vi "DI IRQ BuildMenu.vi"(0 "XRef":T15, 1 "MenuRef":T14, 2 "Point":T13, 3 "Menu Type":T12, 4 "State In":T2) -> (14 "Fatal Error Out":T1)   [LabVIEW 2021, in "myRIO Register DI IRQ.xnode"]
uses:
  <vilib>/myRIO/Instrument Drivers/IRQ/IO IRQ/vis/myRIO Register DI IRQ.xnode
  <vilib>/XNodeSupport/XNodeXNodeRef.ctl
  <vilib>/XNodeSupport/XNodeMenuRef.ctl
  <vilib>/XNodeSupport/XNodePoint.ctl
  <vilib>/XNodeSupport/XNodeInt.ctl
  <vilib>/XNodeSupport/XNodeMenuType.ctl
  <vilib>/myRIO/Instrument Drivers/IRQ/IO IRQ/vis/DI IRQ State.ctl
  <vilib>/myRIO/Common/Instrument Driver Framework/Utilities/typedefs/myRIOXPeripheral.ctl
  <vilib>/XNodeSupport/XNodeTerm4Array.ctl
  <vilib>/XNodeSupport/XNodeTerm4.ctl
  <vilib>/XNodeSupport/XNodeString.ctl
  <vilib>/XNodeSupport/XNodeVariant.ctl
  <vilib>/XNodeSupport/XNodeRect32.ctl
  <vilib>/XNodeSupport/XNodeBool.ctl
  <vilib>/XNodeSupport/XNodeTermDirection.ctl
  <vilib>/XNodeSupport/XNodeErrorCluster.ctl
  <vilib>/XNodeSupport/NI_XNodeSupport.lvlib
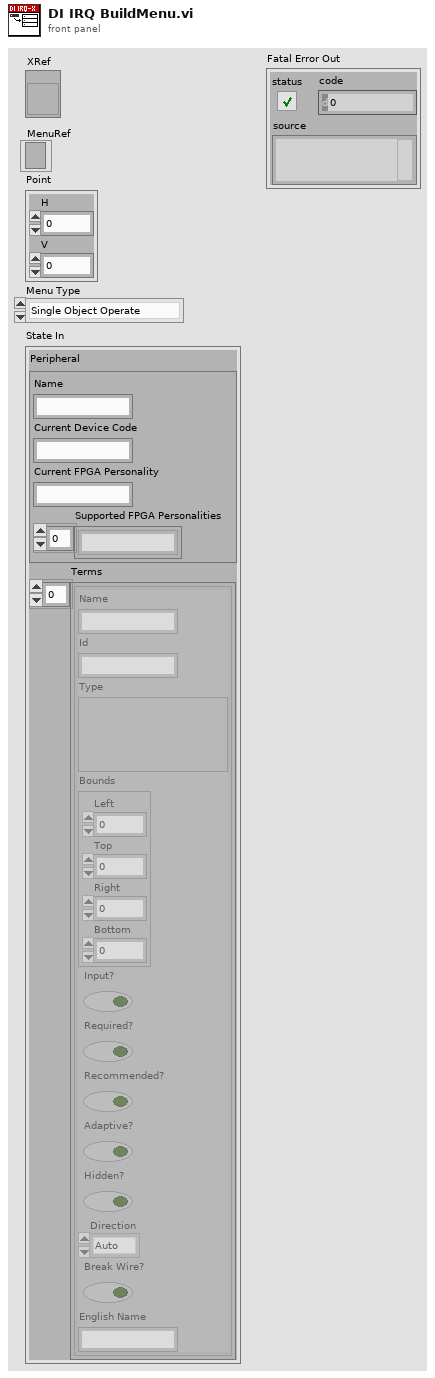
[diagram p1: front panel]
types:
  T1 = typedef "NI_XNodeSupport.lvlib/XNodeErrorCluster.ctl" = errorcluster
  T2 = typedef "myRIO Register DI IRQ.xnode/DI IRQ State.ctl" = cluster{"Peripheral":T3, "Terms":T4}
  T3 = typedef "myRIOXPeripheral.ctl" = cluster{"Name":string, "Current Device Code":string, "Current FPGA Personality":string, "Supported FPGA Personalities":string[]}
  T4 = typedef "NI_XNodeSupport.lvlib/XNodeTerm4Array.ctl" = T5[]
  T5 = typedef "NI_XNodeSupport.lvlib/XNodeTerm4.ctl" = cluster{"Name":T6, "Id":T6, "Type":T7, "Bounds":T8, "Input?":T10, "Required?":T10, "Recommended?":T10, "Adaptive?":T10, "Hidden?":T10, "Direction":T11, "Break Wire?":T10, "English Name":T6}
  T6 = typedef "NI_XNodeSupport.lvlib/XNodeString.ctl" = string
  T7 = typedef "NI_XNodeSupport.lvlib/XNodeVariant.ctl" = variant
  T8 = typedef "NI_XNodeSupport.lvlib/XNodeRect32.ctl" = cluster{"Left":T9, "Top":T9, "Right":T9, "Bottom":T9}
  T9 = typedef "NI_XNodeSupport.lvlib/XNodeInt.ctl" = i32
  T10 = typedef "NI_XNodeSupport.lvlib/XNodeBool.ctl" = bool
  T11 = typedef "NI_XNodeSupport.lvlib/XNodeTermDirection.ctl" = enum32{"Auto", "Up", "Down", "Left", "Right", "Center"}
  T12 = typedef "NI_XNodeSupport.lvlib/XNodeMenuType.ctl" = enum32{"Single Object Operate", "Single Object Popup", "Multi Object Popup Master", "Multi Object Popup Other"}
  T13 = typedef "NI_XNodeSupport.lvlib/XNodePoint.ctl" = cluster{"H":T9, "V":T9}
  T14 = typedef "NI_XNodeSupport.lvlib/XNodeMenuRef.ctl" = refnum<k9>
  T15 = typedef "NI_XNodeSupport.lvlib/XNodeXNodeRef.ctl" = refnum<vi>
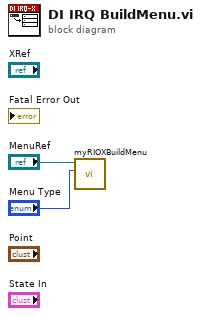
[diagram p0: block diagram]
diagram:
  n1 = call <vilib>:"myRIOXBuildMenu.vi"("Menu Type"="Menu Type", "Menu Reference"="MenuRef") -> ()  [unwired: 9 in, 1 out]
